vi "_Broadcast Message.vi"(7 "Module Pattern (support *)":string, 8 "Error in":errorcluster caption="Error in (no error)", 10 "Argument(\"\")":string, 11 "Broadcast":T1=enum."Macro: Exit") -> (0 "Error out":errorcluster)   [LabVIEW 2017, in "DebugConsole.lvlib"]
uses:
  DebugConsole.lvlib
  _BroadcastDef.ctl
  _csmlite/_csmlite.lvlib
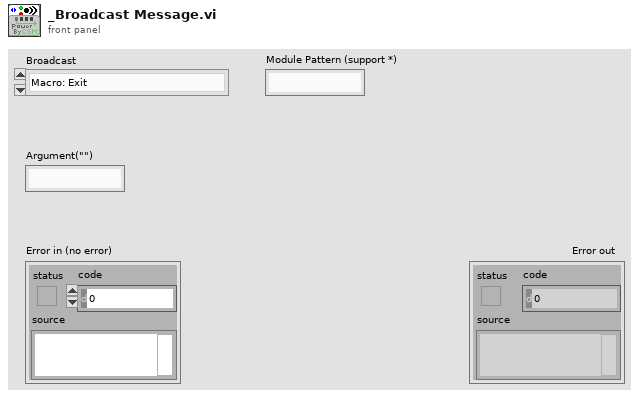
[diagram p1: front panel]
types:
  T1 = typedef "DebugConsole.lvlib/_BroadcastDef.ctl" = enum16{"<no action>", "Macro: Exit", "CSM: Module List Changed", "CSM: Scripts Changed", "CSM: Registration Changed", "CSM: Module Selected", "CSM: Message Excuted", "CSM: Broadcast Excuted", "CSM: Registration Action Excuted", "UI: Try to Change Command"}
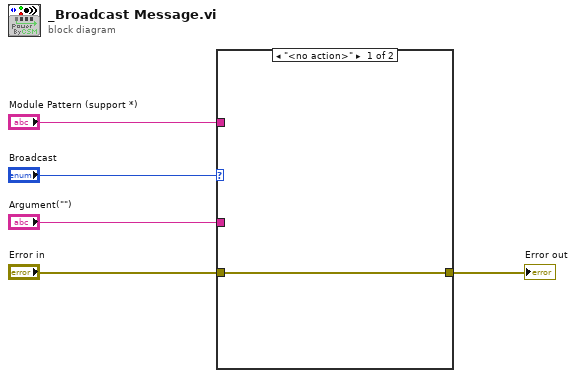
[diagram p0: block diagram]
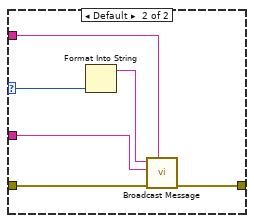
[diagram p2: hidden frame]
diagram:
  n1 = case shown="\"<no action>\"" "Broadcast" {
    selector: "Broadcast" -> [_ w8]
    tunnel: "Module Pattern (support *)" -> [_ w12]
    tunnel: "Error in" -> [w6 w11]
    tunnel: "Argument(\"\")" -> [_ w10]
    tunnel: [w6 w9] -> w2
    frame "<no action>" {
    }
    frame Default {
      n2 = Format Into String(w8) -> (resulting string=w7:string)  [unwired: 3 in, 1 out]
      n3 = call "Broadcast Message.vi"("Module Pattern (support *)"=w12, "Error in"=w11, "Argument(\"\")"=w10, "Message"=w7) -> ("Error out"=w9:errorcluster)  [unwired: 7 in]
    }
  }
  "Error out" <- w2
